vi "Get Signals.vi"(8 "error in (no error)":errorcluster, 11 "Device Item Ref out":T1 format="%.0x") -> (0 "error out":errorcluster, 1 "Parameters":T2[](array[typedef]) {"Byte Order" items=["Little Endian", "Big Endian"]; "Data Type" items=["Signed", "Unsigned", "IEEE Float"]}, 2 "Child Refs":T1[](array[typedef]) format="%.0x", 3 "Item Ref out":T1 format="%.0x")   [LabVIEW 2015, in "Diagnostics Addon System Explorer.lvlib"]
uses:
  System Explorer/Diagnostics Addon System Explorer.lvlib
  <vilib>/NI Veristand/Custom Device API/Custom Device Item Ref.ctl
  Signal Parameters.ctl
  FG Action.ctl
  <vilib>/NI Veristand/Custom Device API/NI VeriStand - Get Item Property.vi
  <vilib>/NI Veristand/Custom Device API/Get Item Property (String).vi
  <vilib>/NI Veristand/Custom Device API/Get Item Property (Double).vi
  <vilib>/NI Veristand/Custom Device API/Get Item Property (U32).vi
  <vilib>/NI Veristand/Custom Device API/NI VeriStand - Set Item Property.vi
  <vilib>/NI Veristand/Custom Device API/Set Item Property (String).vi
  <vilib>/NI Veristand/Custom Device API/Set Item Property (Double).vi
  <vilib>/NI Veristand/Custom Device API/Set Item Property (U32).vi
  GUID Lookup.vi
  <vilib>/NI Veristand/Custom Device API/Custom Device API.lvlib
  Diagnostics Addon Shared.lvlib
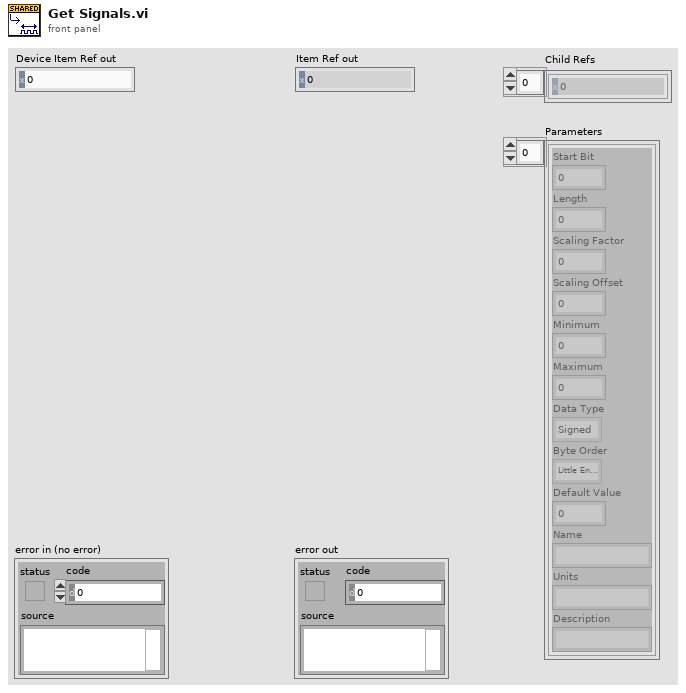
[diagram p1: front panel]
types:
  T1 = typedef "Custom Device API.lvlib/Custom Device Item Ref.ctl" = u64
  T2 = typedef "Diagnostics Addon Shared.lvlib/Signal Parameters.ctl" = cluster{"Start Bit":u8, "Length":u8, "Scaling Factor":dbl, "Scaling Offset":dbl, "Minimum":dbl, "Maximum":dbl, "Data Type":u32, "Byte Order":u32, "Default Value":dbl, "Name":string, "Units":string, "Description":string}
  T3 = typedef "Diagnostics Addon System Explorer.lvlib/FG Action.ctl" = enum16{"Get", "Set"}
  T4 = typedef "Custom Device API.lvlib/Custom Device Channel.ctl" = cluster{"Type":T5, "Units":string, "Default Value":dbl, "Faultable":bool, "Scalable":bool}
  T5 = typedef "Custom Device API.lvlib/Custom Device Channel Type.ctl" = enum16{"Input", "Output"}
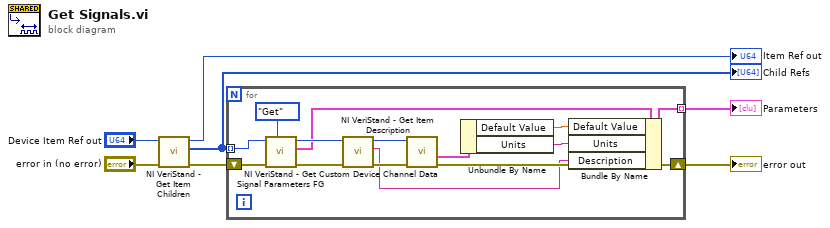
[diagram p0: block diagram]
diagram:
  n1 = call <vilib>:"NI VeriStand - Get Item Children.vi"("error in (no error)"="error in (no error)", "Item Ref in"="Device Item Ref out") -> ("error out"=w2:errorcluster, "Child Refs"=w3:T1[], "Item Ref out"=→"Item Ref out":T1)  [unwired: 6 in, 1 out]
  "Child Refs" <- w3
  n2 = for {
    shift-right: [w19] -> w7
    shift-left: w2 -> [w21]
    tunnel: w3 -> [w20] mode=indexing
    tunnel: [w16] -> w1 mode=indexing
    n3 = call "Signal Parameters FG.vi"("Action"=FG_Action."Get", "error in (no error)"=w21, "Device Item Ref in"=w20) -> ("error out"=w10:errorcluster, "Signal Parameters"=w17:T2, "Device Item Ref out"=w18:T1)  [unwired: 6 in]
    n4 = call <vilib>:"NI VeriStand - Get Item Description.vi"("error in (no error)"=w10, "Item Ref in"=w18) -> ("error out"=w11:errorcluster, "Description"=w9:string, "Item Ref out"=w12:T1)  [unwired: 6 in, 1 out]
    n5 = call <vilib>:"NI VeriStand - Get Custom Device Channel Data.vi"("error in (no error)"=w11, "Channel Ref in"=w12) -> ("error out"=w19:errorcluster, "Channel"=w15:T4)  [unwired: 4 in, 4 out]
    n6 = Unbundle By Name(w15) -> ("Default Value"=w13:dbl, "Units"=w14:string)
    n7 = Bundle By Name(cluster=w17, "Default Value"=w13, "Units"=w14, "Description"=w9) -> (w16:T2)
  }
  "error out" <- w7
  "Parameters" <- w1
